vi "stubs.vi"() -> ()   [LabVIEW 2015]
uses:
  <vilib>/rvi/interface/nirviMethod/nirviMethod.xnode
  <vilib>/rvi/interface/nirviMethod/StockFPGA_InlinedMethodWaitForSingleIRQ.vi
  <vilib>/FPGAPlugInAG/Dynamic/niLvFpga_WaitOnIrq_Dynamic.vi
  <vilib>/FPGAPlugInAG/Dynamic/niLvFpga_AcknowledgeIrq_Dynamic.vi
panel:
  in  "Stop System (Careful!!)":bool
  out "Test Loop iterator":i32
  in  "path":path
  out "path out":path
  out "filenames":string[](array[string])
  out "folder names":string[](array[string])
  out "test error out":errorcluster
  in  "pattern":string
  in  "Test":bool
  out "Testing":bool
  out "IRQ Timed Out":bool
  in  "IRQ Timeout (ms)":i32=10000
  out "Wait Until Cleared":bool
  in  "Interrupt Boolean":bool
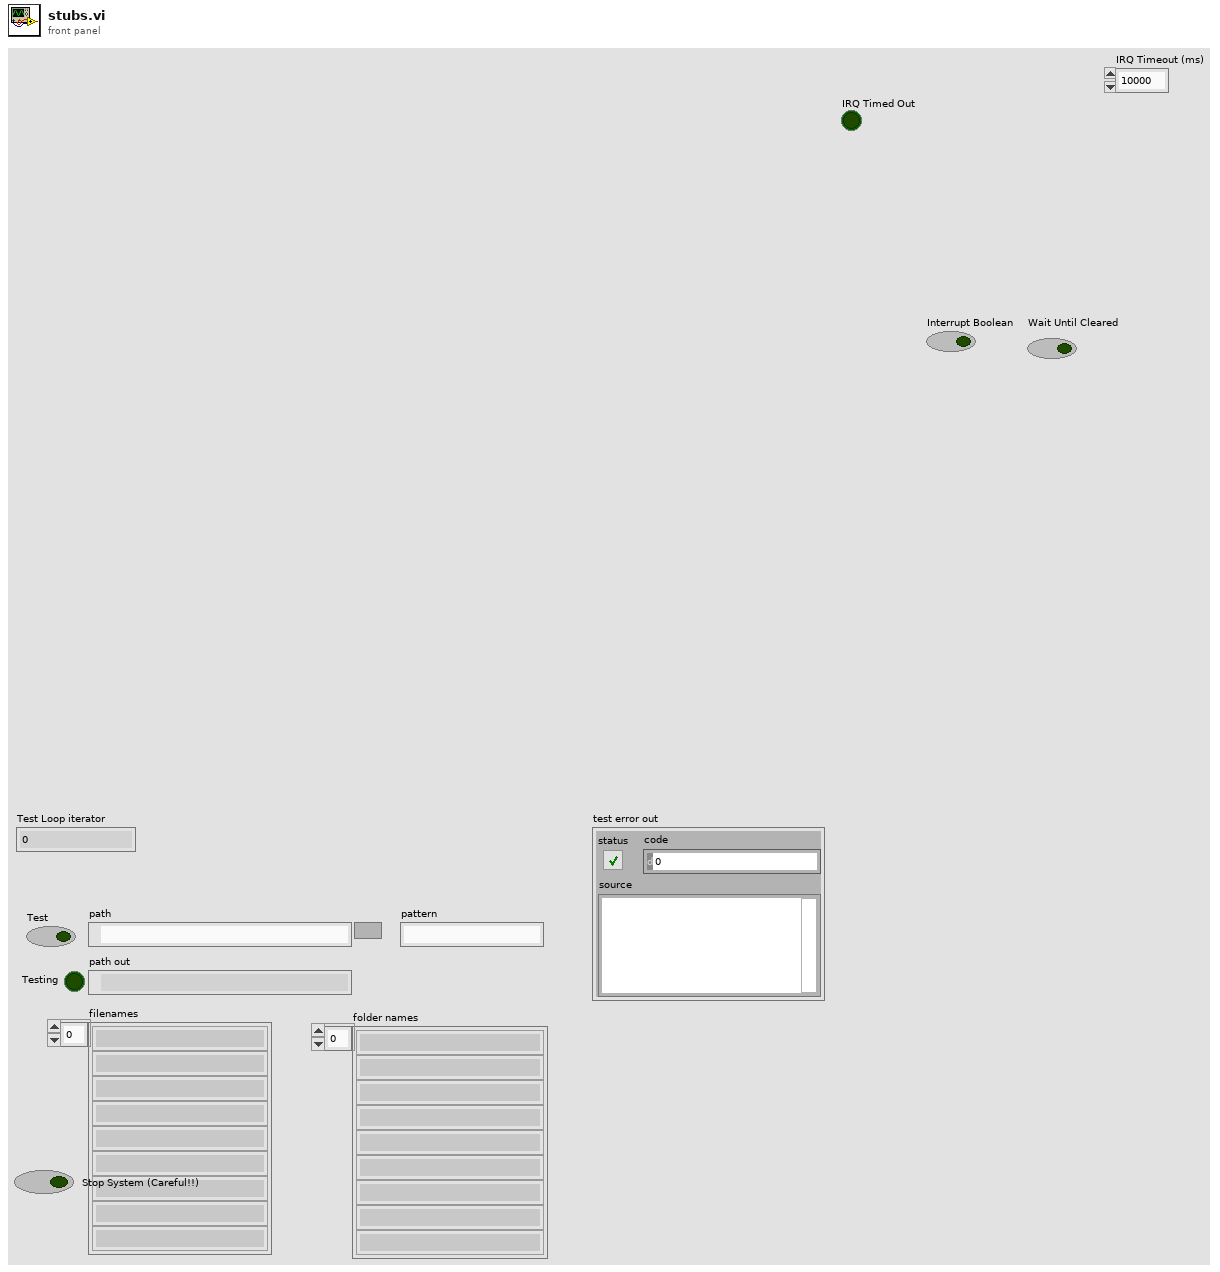
[diagram p1: front panel]
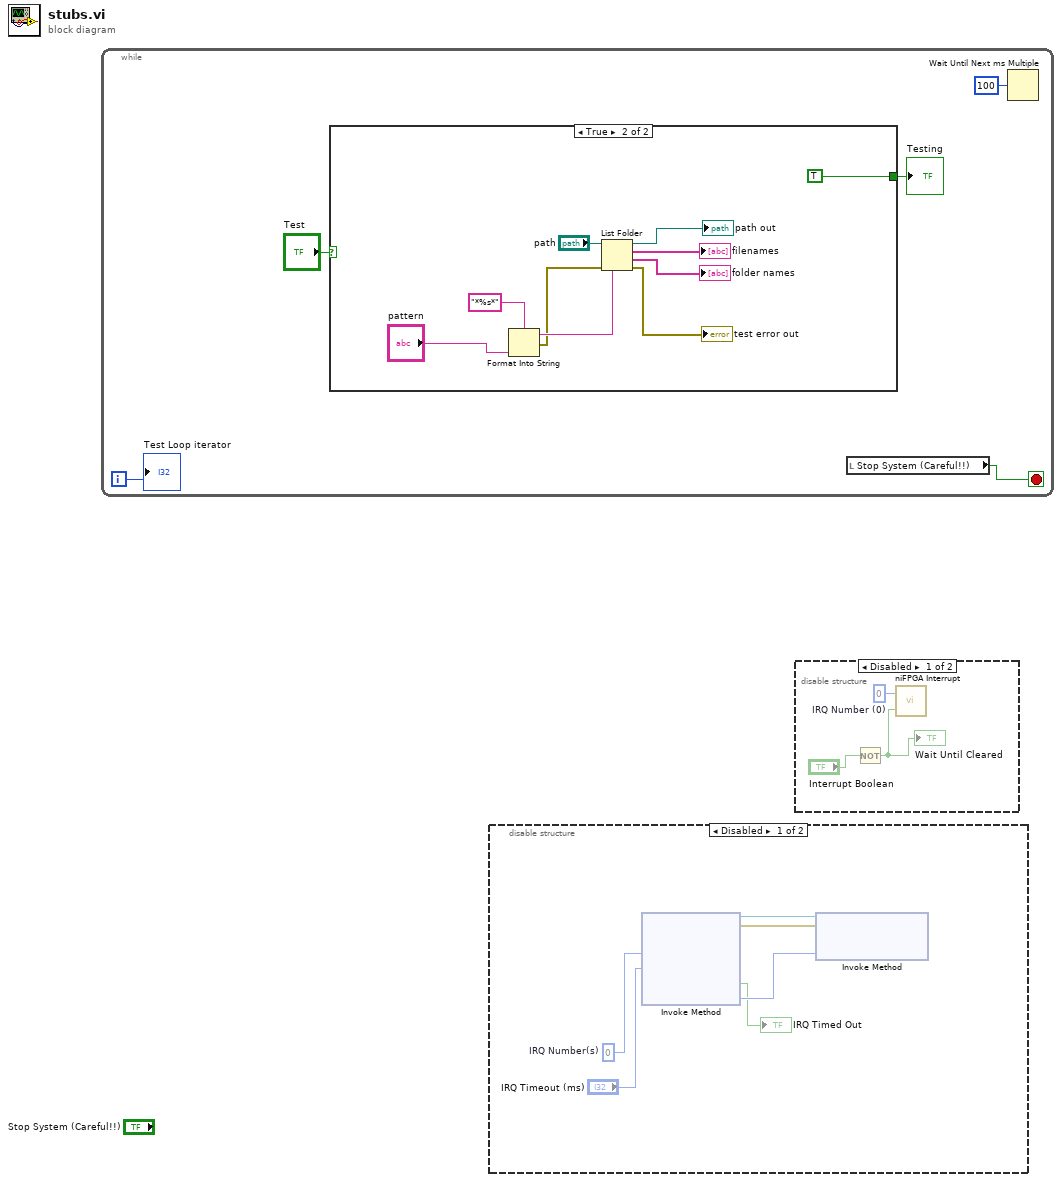
[diagram p0: block diagram]
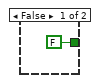
[diagram p2: hidden frame]
diagram:
  n1 = while {
    i -> [w3]
    stop <- w5 stop-if-true
    n2 = case shown="True" "Test" {
      tunnel: [FALSE TRUE] -> w1
      frame False {
      }
      frame True {
        n3 = Format Into String(format string="*%s*", "pattern") -> (resulting string=w8:string, error out=w7:errorcluster)  [unwired: 2 in]
        n4 = List Folder(path="path", pattern=w8, error in=w7) -> (path out=→"path out":path, filenames=→"filenames":string[], folder names=→"folder names":string[], error out=→"test error out":errorcluster)  [unwired: 1 in]
      }
    }
    "Testing" <- w1
    n5 = local read "Stop System (Careful!!)"() -> (w5:bool)
    n6 = Wait Until Next ms Multiple(millisecond multiple=u32 100) -> ()  [unwired: 1 out]
    "Test Loop iterator" <- w3
  }
  n7 = disable-structure shown="Disabled" {
    frame Disabled {
      w20 = 0  # IRQ Number(s)
      n8 = xnode "Invoke Method"("IRQ Number(s)"=w20, "Timeout (ms)"="IRQ Timeout (ms)") -> ("FPGA VI Reference Out"=w18:refnum<k20>, "error out"=w17:errorcluster, "Timed Out"=→"IRQ Timed Out":bool, "IRQ(s) Asserted"=w22:i32)  [unwired: 2 in]
      n9 = xnode "Invoke Method"("FPGA VI Reference In"=w18, "error in"=w17, "IRQ Number(s)"=w22) -> ()  [unwired: 2 out]
    }
    frame Enabled {
    }
  }
  n10 = disable-structure shown="Disabled" {
    frame Disabled {
      w25 = u8 0  # IRQ Number (0)
      n11 = Not(x="Interrupt Boolean") -> (.not. x?=w24:bool)
      "Wait Until Cleared" <- w24
      n12 = call <vilib>:"niFPGA Interrupt.vi"("Wait Until Cleared (F)"=w24, "IRQ Number (0)"=w25) -> ()  [unwired: 1 in]
    }
    frame Enabled {
    }
  }
